vi "WSVCAP SHL FPGA LL RFFE FIFO Manager - Transfer.vi"(9 "Word In":u64, 11 "error in (no error)":errorcluster, 13 "Operation":T1) -> (4 "Data Out":u64, 8 "Timed Out":bool, 15 "error out":errorcluster)   [LabVIEW 2017]
uses:
  Type Defs/WSVCAP SHL FIFO Operation Enum.ctl
  <vilib>/rvi/Emulation/niFpgaProcessEmulError.vi
  <vilib>/rvi/DataTransferAndStorage/Container/Common/niFpgaContainerGetUniqueNameForEmu.vi
  <vilib>/rvi/FIFO/Fifo_Resource/nirvififoEmulationSetSize.vi
  <vilib>/rvi/FIFO/Fifo_Resource/nirviFifoEmulationQueueMgr.vi
  <instcachedir>/0/nirviFifoEmulationQueueMgr_E5CAEC123FF24DC58D834DCA3CDAA9B5.lvgen/nirviFifoEmulationQueueMgr_E5CAEC123FF24DC58D834DCA3CDAA9B5_001.vi
  <vilib>/rvi/Emulation/niFpgaEmulationIsFPGAContextNoSignature.vi
  <vilib>/rvi/eio/common/nirviEmuReportErrorAndStop.vi
  <vilib>/rvi/errors/nirviReportUnexpectedCaseInternalError.vi
  <vilib>/rvi/errors/nirviReportUnexpectedCaseInternalError (U32).vi
  <vilib>/rvi/occurrence/nirviWaitOnOccurrenceBase.vi
  <vilib>/rvi/FIFO/Fifo_Resource/nirvififoEmulationReleaseLock.vi
  <vilib>/rvi/FIFO/Fifo_Resource/nirvififoEmulationObtainLock.vi
  <vilib>/rvi/FIFO/Fifo_Resource/nirvififoEmulationCreateLock.vi
  <vilib>/Utility/error.llb/Clear Errors.vi
  <instcachedir>/0/nirviFifoEmulationQueueMgr_E5CAEC123FF24DC58D834DCA3CDAA9B5.lvgen/nirviFifoEmulationQueueMgr_E5CAEC123FF24DC58D834DCA3CDAA9B5_002.vi
  <vilib>/rvi/errors/niFpgaSetErrorForExecOnDevCompSimple.vi
  <vilib>/rvi/Emulation/niFpgaSctlEmulationGetInTimedLoop.vi
  <vilib>/rvi/FIFO/Fifo_Resource/nirvififoEmulationDetermineInputValidOut.vi
  <vilib>/rvi/DataTransferAndStorage/Container/XNode/niFpgaContainer.xnode
  <vilib>/rvi/FIFO/Fifo_Resource/nirvififoEmulationGetNumberOfElementsToRead.vi
  <vilib>/rvi/FIFO/Fifo_Resource/nirvififoEmulationRead.vi
  <vilib>/rvi/FIFO/Fifo_Resource/nirvififoEmulationWrite.vi
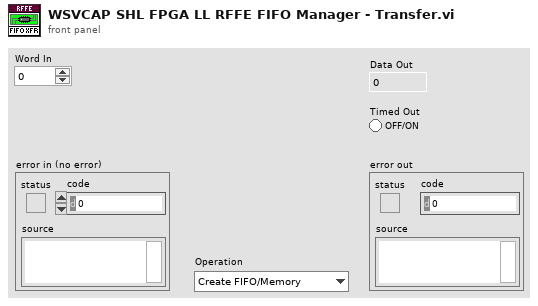
[diagram p1: front panel]
types:
  T1 = typedef "WSVCAP SHL FIFO Operation Enum.ctl" = enum16{"Create FIFO/Memory", "Get Write FIFO Status", "Get Read FIFO Status", "Put Element in Write", "Put Element in Read", "Get Element from Write", "Get Element from Read"}
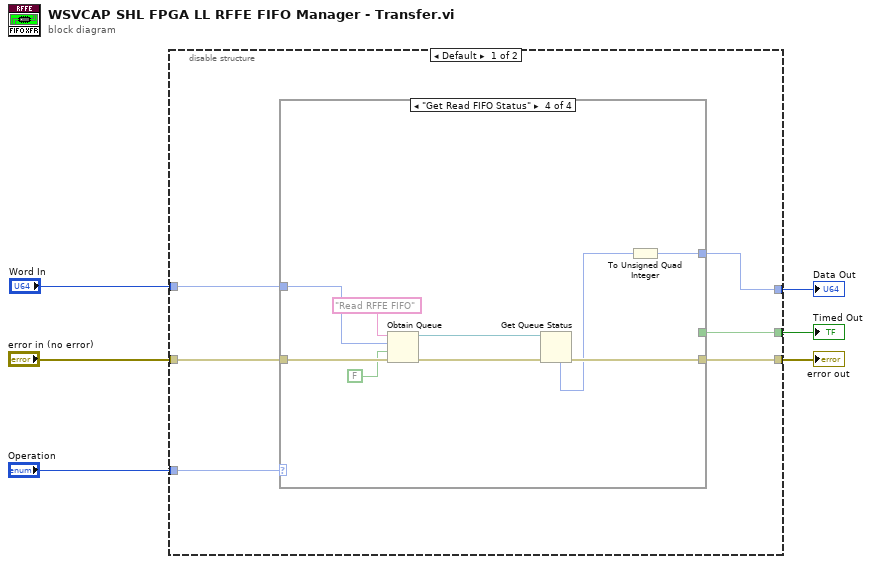
[diagram p0: block diagram]
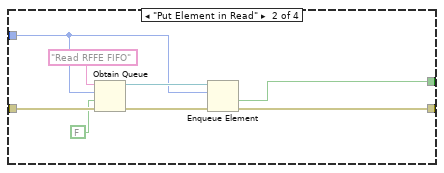
[diagram p3: hidden frame]
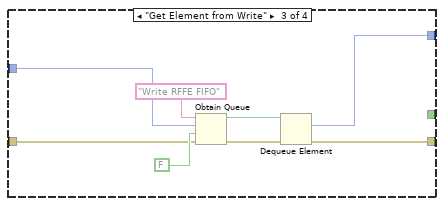
[diagram p4: hidden frame]
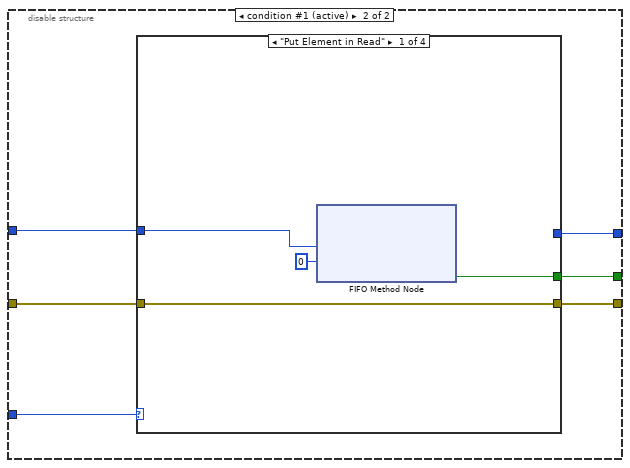
[diagram p5: hidden frame]
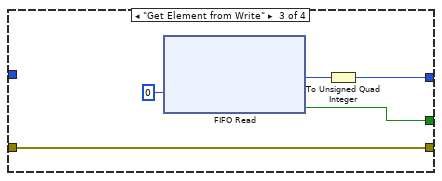
[diagram p7: hidden frame]
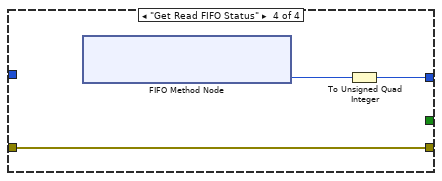
[diagram p8: hidden frame]
diagram:
  n1 = disable-structure shown="Default" {
    disable-tunnel: "Operation" -> [w12 w44]
    disable-tunnel: "error in (no error)" -> [w11 w42]
    disable-tunnel: [w10 w41] -> w4
    disable-tunnel: [w9 w40] -> w1
    disable-tunnel: [w8 w43] -> w3
    disable-tunnel: "Word In" -> [w7 w39]
    frame condition #0 {
      n2 = case shown="\"Get Read FIFO Status\"" w12 {
        tunnel: [w13 w21 w24 w38] -> w10
        tunnel: w11 -> [w13 w19 w25 w37]
        tunnel: [_ _ w22 w30] -> w9
        tunnel: [_ w20 _ _] -> w8
        tunnel: w7 -> [_ w14 w23 w34]
        frame Default {
        }
        frame "Put Element in Read" {
          n3 = Obtain Queue(name (unnamed)="Read RFFE FIFO", element data type=w14, create if not found? (T)=FALSE, error in (no error)=w19) -> (queue out=w17:refnum<queue>, error out=w18:errorcluster)  [unwired: 1 in, 1 out]
          n4 = Enqueue Element(queue=w17, element=w14, error in (no error)=w18) -> (timed out?=w20:bool, error out=w21:errorcluster)  [unwired: 1 in, 1 out]
        }
        frame "Get Element from Write" {
          n5 = Obtain Queue(name (unnamed)="Write RFFE FIFO", element data type=w23, create if not found? (T)=FALSE, error in (no error)=w25) -> (queue out=w27:refnum<queue>, error out=w29:errorcluster)  [unwired: 1 in, 1 out]
          n6 = Dequeue Element(queue=w27, error in (no error)=w29) -> (element=w22:u64, error out=w24:errorcluster)  [unwired: 1 in, 2 out]
        }
        frame "Get Read FIFO Status" {
          n7 = Obtain Queue(name (unnamed)="Read RFFE FIFO", element data type=w34, create if not found? (T)=FALSE, error in (no error)=w37) -> (queue out=w33:refnum<queue>, error out=w32:errorcluster)  [unwired: 1 in, 1 out]
          n8 = Get Queue Status(queue=w33, error in (no error)=w32) -> (error out=w38:errorcluster, # elements in queue=w31:i32)  [unwired: 1 in, 6 out]
          n9 = To Unsigned Quad Integer(1:w31) -> (0:w30:u64)
        }
      }
    }
    frame condition #1 (active) {
      n10 = case shown="\"Put Element in Read\"" w44 {
        tunnel: [w47 _ w51 _] -> w43
        tunnel: w42 -> [w48 w49 w54 w57]
        tunnel: [w48 w49 w54 w57] -> w41
        tunnel: [_ _ w50 w55] -> w40
        tunnel: w39 -> [w45 _ _ _]
        frame "Put Element in Read" {
          n11 = xnode ("FIFO Method Node")("Element"=w45, "Timeout"=0) -> ("Timed Out?"=w47:bool)  [unwired: 2 in, 2 out]
        }
        frame Default {
        }
        frame "Get Element from Write" {
          n12 = xnode "FIFO Read"("Timeout"=0) -> ("Element"=w53:u16, "Timed Out?"=w51:bool)  [unwired: 1 in, 1 out]
          n13 = To Unsigned Quad Integer(1:w53) -> (0:w50:u64)
        }
        frame "Get Read FIFO Status" {
          n14 = xnode ("FIFO Method Node")() -> ("Number of Elements to Read"=w56:u32)  [unwired: 2 in, 2 out]
          n15 = To Unsigned Quad Integer(1:w56) -> (0:w55:u64)
        }
      }
    }
  }
  "error out" <- w4
  "Timed Out" <- w3
  "Data Out" <- w1
